vi "Actor Core.vi"(8 "error in":errorcluster, 11 "Settings in":refnum<class "Settings.lvclass">) -> (0 "error out":errorcluster, 3 "Actor out":refnum<class "Actor.lvclass">)   [LabVIEW 2015, in "Item Actor.lvlib" / "Settings.lvclass"]
doc: "(<B>Filename</B>: Actor Framework.lvlib:Actor.lvclass:Actor Core.vi)\n\nReceives messages to the actor, reacts to them, and initiates any error handling that may shut the actor down.\n\nDescendant classes may override this VI to append parallel tasks for the actor to complete while it handles messages. Overrides use the Call Parent Method node."
uses:
  Settings.lvclass
  <vilib>/ActorFramework/Actor/Actor.lvclass
  Settings.lvclass/Settings.ctl
  <vilib>/ActorFramework/Actor/Actor.lvclass/Actor.ctl
  <vilib>/ActorFramework/Message Enqueuer/Message Enqueuer.lvclass/Message Enqueuer.ctl
  VI Store/VIStore Messages/Register Settings Changes Msg/Register Settings Changes Msg.lvclass/Register Settings Changes Msg.ctl
  <vilib>/ActorFramework/Message Enqueuer/Init from Existing Queue.vi
  <vilib>/ActorFramework/Message Enqueuer/Enqueue.vi
  <vilib>/ActorFramework/Message Priority Queue/Priority Enqueue.vi
  <vilib>/ActorFramework/Message Enqueuer/Message Enqueuer.lvclass
  <vilib>/ActorFramework/Stop Msg/Stop Msg.lvclass
  VI Store/VIStore Messages/Register Settings Changes Msg/Register Settings Changes Msg.lvclass
  Generic Item/Generic Item.lvclass
  VI Store/VIStore Actor/VIStore.lvclass
panel:
  in  "Resizable":bool
  in  "Instruments Repository":path
  in  "Apply":bool
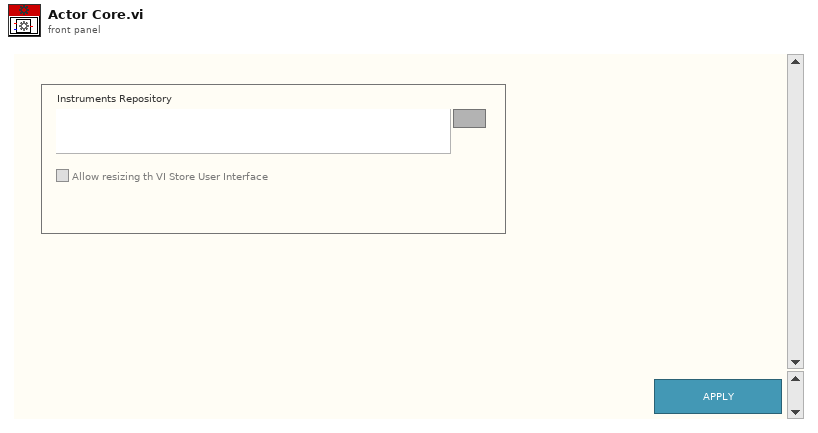
[diagram p1: front panel]
types:
  T1 = enum8{"Enabled", "Disabled", "Disabled and Grayed Out"}
  T2 = typedef "Item Actor.lvlib/Settings.lvclass/Settings Data.ctl" = cluster{"Categories Path":path, "Resizable":bool}
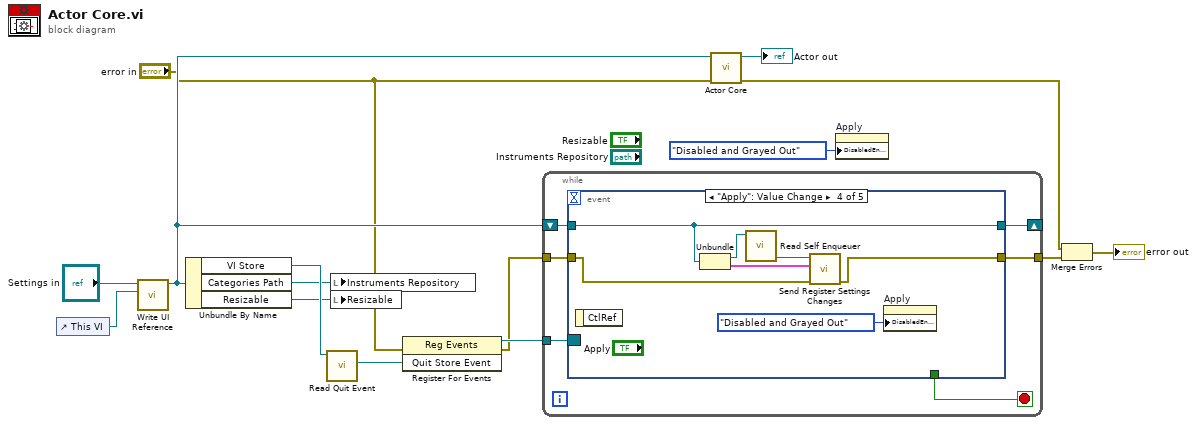
[diagram p0: block diagram]
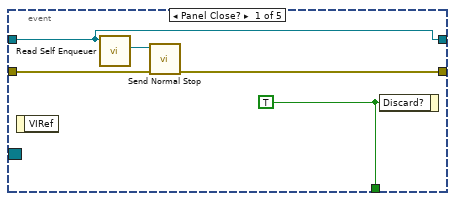
[diagram p2: hidden frame]
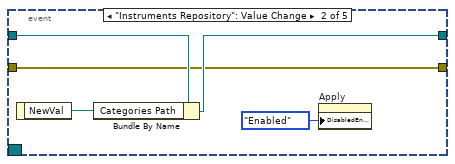
[diagram p3: hidden frame]
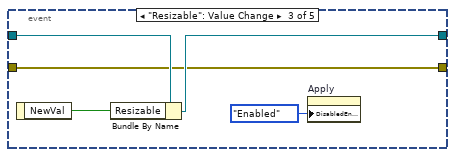
[diagram p4: hidden frame]
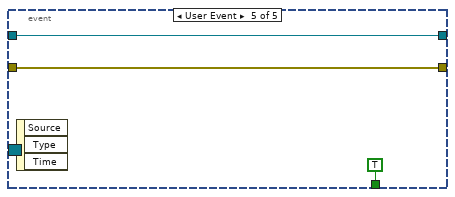
[diagram p5: hidden frame]
diagram:
  n1 = control-ref of="This VI"() -> (w14:refnum<vi>)
  n2 = call "Write UI Reference.vi"("Item Panel"=w14, "Generic Item in"="Settings in") -> ("Generic Item out"=w11:refnum<class "Settings.lvclass">)  [unwired: 8 in, 1 out]
  n3 = Unbundle By Name(w11) -> ("VI Store"=w10:refnum<class "VIStore.lvclass">, "Categories Path"=w7:path, "Resizable"=w6:bool)
  n4 = call "Read Quit Event.vi"("VIStore in"=w10) -> ("Quit Store Event"=w9:refnum<user-event>)  [unwired: 8 in, 2 out]
  n5 = local write "Instruments Repository"(w7) -> ()
  n6 = local write "Resizable"(w6) -> ()
  n7 = register-events(error in="error in", w9) -> (reference out=w8:refnum<event-registration>, error out=w4:errorcluster)  [unwired: 1 in]
  n8 = while {
    shift-right: [w19] -> _
    shift-left: w11 -> [w21]
    tunnel: w8 -> [w18]
    tunnel: w4 -> [w17]
    tunnel: [w16] -> w3
    stop <- w20 stop-if-true
    n9 = event shown="[3] \"Apply\": Value Change" {
      selector: w18 -> [_ _ _ _ _]
      dyn-events: _ -> [_ _ _ _ _]
      timeout: _ -> [_ _ _ _ _]
      tunnel: w21 -> [w24 w31 w36 w40 w45]
      tunnel: [w26 _ _ _ TRUE ("Discard?")] -> w20
      tunnel: [w24 w29 w34 w40 w45] -> w19
      tunnel: w17 -> [w23 w27 w32 w38 w44]
      tunnel: [w22 w27 w32 w37 w44] -> w16
      event Panel Close? {
        w26 = TRUE ("Discard?")
        n10 = event-data() -> ()  [unwired: 1 in, 1 out]
        n11 = call <vilib>:"Read Self Enqueuer.vi"("Actor"=w24) -> ("Self Enqueuer"=w25:refnum<class "Message Enqueuer.lvclass">)  [unwired: 10 in]
        n12 = call <vilib>:"Send Normal Stop.vi"("error in (no error)"=w23, "Message Enqueuer"=w25) -> ("error out"=w22:errorcluster)  [unwired: 9 in]
        n13 = event-data("Discard?"=w26) -> ()  [unwired: 1 in, 1 out]
      }
      event "Instruments Repository": Value Change {
        n14 = event-data() -> ("NewVal"=w30:path)  [unwired: 1 in]
        n15 = Bundle By Name(cluster=w31, "Categories Path"=w30) -> (w29:refnum<class "Settings.lvclass">)
        n16 = property on="Apply" class="Bool"("DisabledEnum"=T1."Enabled" ("Disabled")) -> ()  [unwired: 2 in, 2 out]
      }
      event "Resizable": Value Change {
        n17 = event-data() -> ("NewVal"=w35:bool)  [unwired: 1 in]
        n18 = Bundle By Name(cluster=w36, "Resizable"=w35) -> (w34:refnum<class "Settings.lvclass">)
        n19 = property on="Apply" class="Bool"("DisabledEnum"=T1."Enabled" ("Disabled")) -> ()  [unwired: 2 in, 2 out]
      }
      event "Apply": Value Change {
        n20 = event-data() -> ()  [unwired: 1 in, 1 out]
        n21 = Unbundle(w40) -> (w43:refnum<class "VIStore.lvclass">, w41:T2)
        n22 = call <vilib>:"Read Self Enqueuer.vi"("Actor"=w43) -> ("Self Enqueuer"=w42:refnum<class "Message Enqueuer.lvclass">)  [unwired: 10 in]
        n23 = call "Send Register Settings Changes.vi"("error in (no error)"=w38, "Settings Data"=w41, "Message Enqueuer"=w42) -> ("error out"=w37:errorcluster)  [unwired: 7 in, 1 out]
        n24 = property on="Apply" class="Bool"("DisabledEnum"=T1."Disabled and Grayed Out" ("Disabled")) -> ()  [unwired: 2 in, 2 out]
      }
      event User Event {
        n25 = event-data() -> ()  [unwired: 1 in, 3 out]
      }
    }
  }
  n26 = call-parent "Actor Core.vi"("error in"="error in", "Generic Item in"=w11) -> ("error out"=w2:errorcluster, "Actor out"=→"Actor out":refnum<class "Actor.lvclass">)  [unwired: 8 in]
  n27 = property on="Apply" class="Bool"("DisabledEnum"=T1."Disabled and Grayed Out" ("Disabled")) -> ()  [unwired: 2 in, 2 out]
  n28 = Merge Errors(w2, w3) -> (→"error out":errorcluster)
